vi "Write Parameters.vi"(8 "error in (no error)":errorcluster, 10 "Parameters table VCH":u32[](array[numeric])=[0, 10000, 5000, 1000, 0, 2], 11 "valve_VCH in":refnum<class "valve_VCH.lvclass">) -> (0 "error out":errorcluster, 3 "valve_VCH out":refnum<class "valve_VCH.lvclass">)   [LabVIEW 2019, in "valve_VCH.lvclass"]
uses:
  valve_VCH.lvclass
  valve_VCH.lvclass/valve_VCH.ctl
  Z_state/valve_VCH_Z_state.lvclass/valve_VCH_Z_state.ctl
  ZM_state/valve_VCH_ZM_state.lvclass/valve_VCH_ZM_state.ctl
  Z_state/valve_VCH_Z_state.lvclass
  ZM_state/valve_VCH_ZM_state.lvclass
panel:
  # "0 - T_start_delay\n1 - T_check\n2 - T_big_pause\n3 - T_little_pause\n4 - T_impuls\n5 - N_repeat"
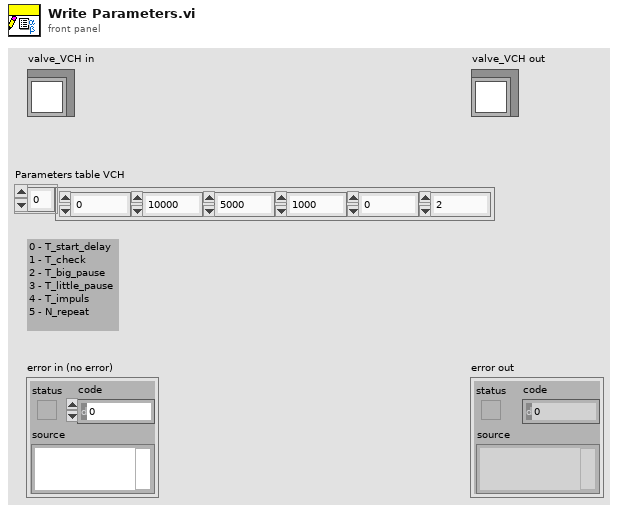
[diagram p1: front panel]
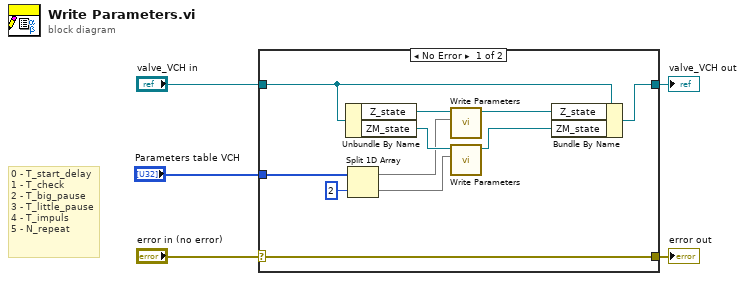
[diagram p0: block diagram]
diagram:
  # "0 - T_start_delay\n1 - T_check\n2 - T_big_pause\n3 - T_little_pause\n4 - T_impuls\n5 - N_repeat"
  n1 = case shown="No Error" "error in (no error)" {
    selector: "error in (no error)" -> [w16 w17]
    tunnel: [w16 w17] -> w4
    tunnel: [w15 w18] -> w2
    tunnel: "valve_VCH in" -> [w14 w18]
    tunnel: "Parameters table VCH" -> [w10 _]
    frame No Error {
      n2 = Unbundle By Name(w14) -> ("Z_state"=w13:refnum<class "valve_VCH_Z_state.lvclass">, "ZM_state"=w12:refnum<class "valve_VCH_ZM_state.lvclass">)
      n3 = Split 1D Array(array=w10, index=2) -> (first subarray=w9:u32[], second subarray=w8:u32[])
      n4 = call "Write Parameters.vi"("Parameters"=w9, "valve_VCH_Z_state in"=w13) -> ("valve_VCH_Z_state out"=w7:refnum<class "valve_VCH_Z_state.lvclass">)  [unwired: 9 in]
      n5 = call "Write Parameters.vi"("Parameters"=w8, "valve_VCH_ZM_state in"=w12) -> ("valve_VCH_ZM_state out"=w6:refnum<class "valve_VCH_ZM_state.lvclass">)  [unwired: 9 in]
      n6 = Bundle By Name(cluster=w14, "Z_state"=w7, "ZM_state"=w6) -> (w15:refnum<class "valve_VCH.lvclass">)
    }
    frame Error {
    }
  }
  "error out" <- w4
  "valve_VCH out" <- w2
